vi "Add Result Column Width.vi"(8 "Result index":i32, 11 "Relative Column Widths (%)":sgl[](array[numeric])) -> (3 "Relative Column Widths (%) out":sgl[](array[numeric]))   [LabVIEW 2020, in "PDF Interface.lvlib" / "PDF Interface Helper.lvlib"]
uses:
  PDF Interface Helper.lvlib
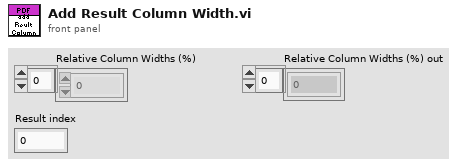
[diagram p1: front panel]
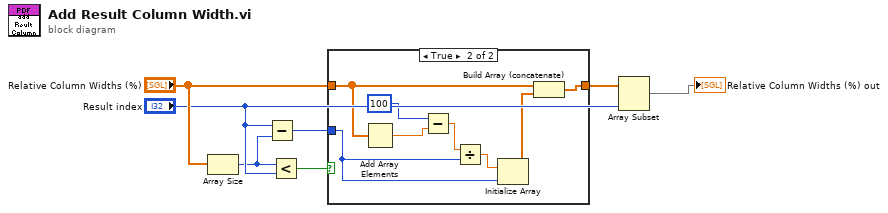
[diagram p0: block diagram]
diagram:
  n1 = Array Size(array="Relative Column Widths (%)") -> (size(s)=w2:i32)
  n2 = Subtract(x="Result index", y=w2) -> (x-y=w1:i32)
  n3 = Less?(x=w2, y="Result index") -> (x < y?=w6:bool)
  n4 = case shown="True" w6 {
    tunnel: [w8 w13] -> w5
    tunnel: "Relative Column Widths (%)" -> [w8 w14]
    tunnel: w1 -> [_ w10]
    frame False {
    }
    frame True {
      n5 = Add Array Elements(numeric array=w14) -> (sum=w15:sgl)
      n6 = Subtract(x=100, y=w15) -> (x-y=w12:sgl)
      n7 = Divide(x=w12, y=w10) -> (x/y=w11:sgl)
      n8 = Initialize Array(w11, w10) -> (w9:sgl[])
      n9 = Build Array (concatenate)(w14, w9) -> (w13:sgl[])
    }
  }
  n10 = Array Subset(array=w5, length="Result index") -> (→"Relative Column Widths (%) out":sgl[])  [unwired: 1 in]
